vi "resonant.image queue to disk and to display queue_MD.vi"() -> ()   [LabVIEW 2012]
uses:
  <vilib>/Utility/VariantDataType/Type.ctl
  Custom Controls/file format type def.ctl
  GFG/GFGnumericGet.vi
  GFG/GFGbooleanGet.vi
  GFG/GFGstringGet.vi
  save images/save channels to raw bin files.vi
  save images/save channels to interleaved multi-tiff files.vi
  save images/save channels to separate multi-tiff files.vi
  save images/save channels to stacked multi-tiff files.vi
  save images/save channels to interleaved tiff series.vi
  save images/save channels to separate tiff series.vi
  save images/save channels to stacked tiff series.vi
  GFG/GFG library.lvlib
  <vilib>/Utility/VariantDataType/VariantType.lvlib
panel:
  out "element":i32
  out "error out 5":errorcluster
  out "size(s)":i32[](array[numeric])
  out "x/y":dbl
  out "error out 4":errorcluster
  out "error out 3":errorcluster
  out "error out 2":errorcluster
  out "# elements in image data queue":i32
  out "error out":errorcluster
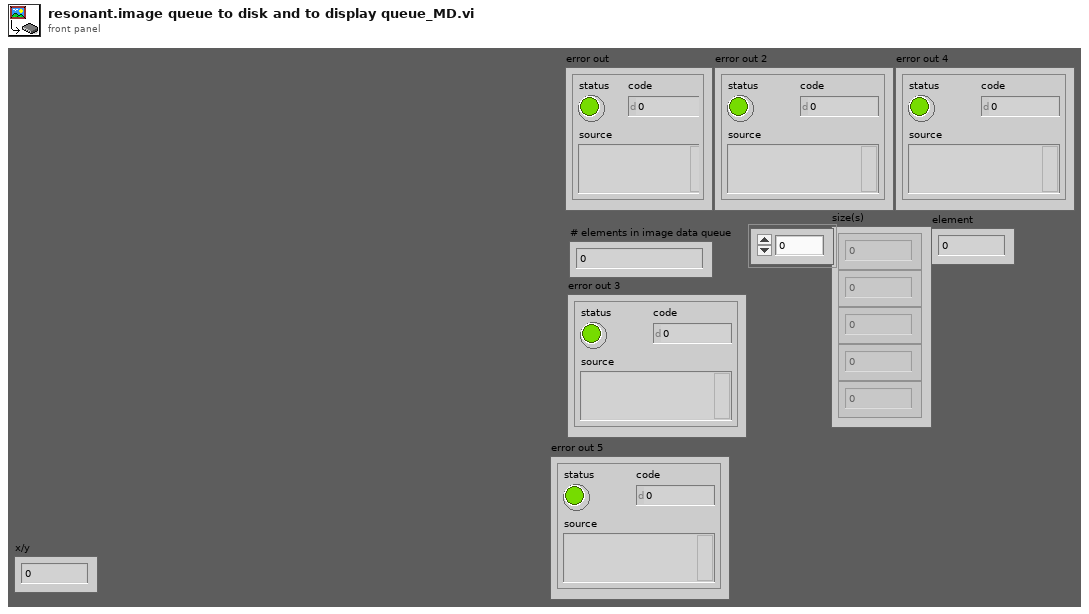
[diagram p1: front panel]
types:
  T1 = typedef "file format type def.ctl" = enum16{"16bit raw", "32bit raw", "16bit multi-tiff (interleave)", "16bit multi-tiff (separate)", "16bit multi-tiff (stacked)", "32bit multi-tiff (interleave)", "32bit multi-tiff (separate)", "32bit multi-tiff (stacked)", "16bit tiff series (interleave)", "16bit tiff series (separate)", "16bit tiff series (stacked)", "32bit tiff series (interleave)", "32bit tiff series (separate)", "32bit tiff series (stacked)"}
  T2 = cluster{"NewVal":bool, "Event Registration Refnum":refnum<event-registration>}
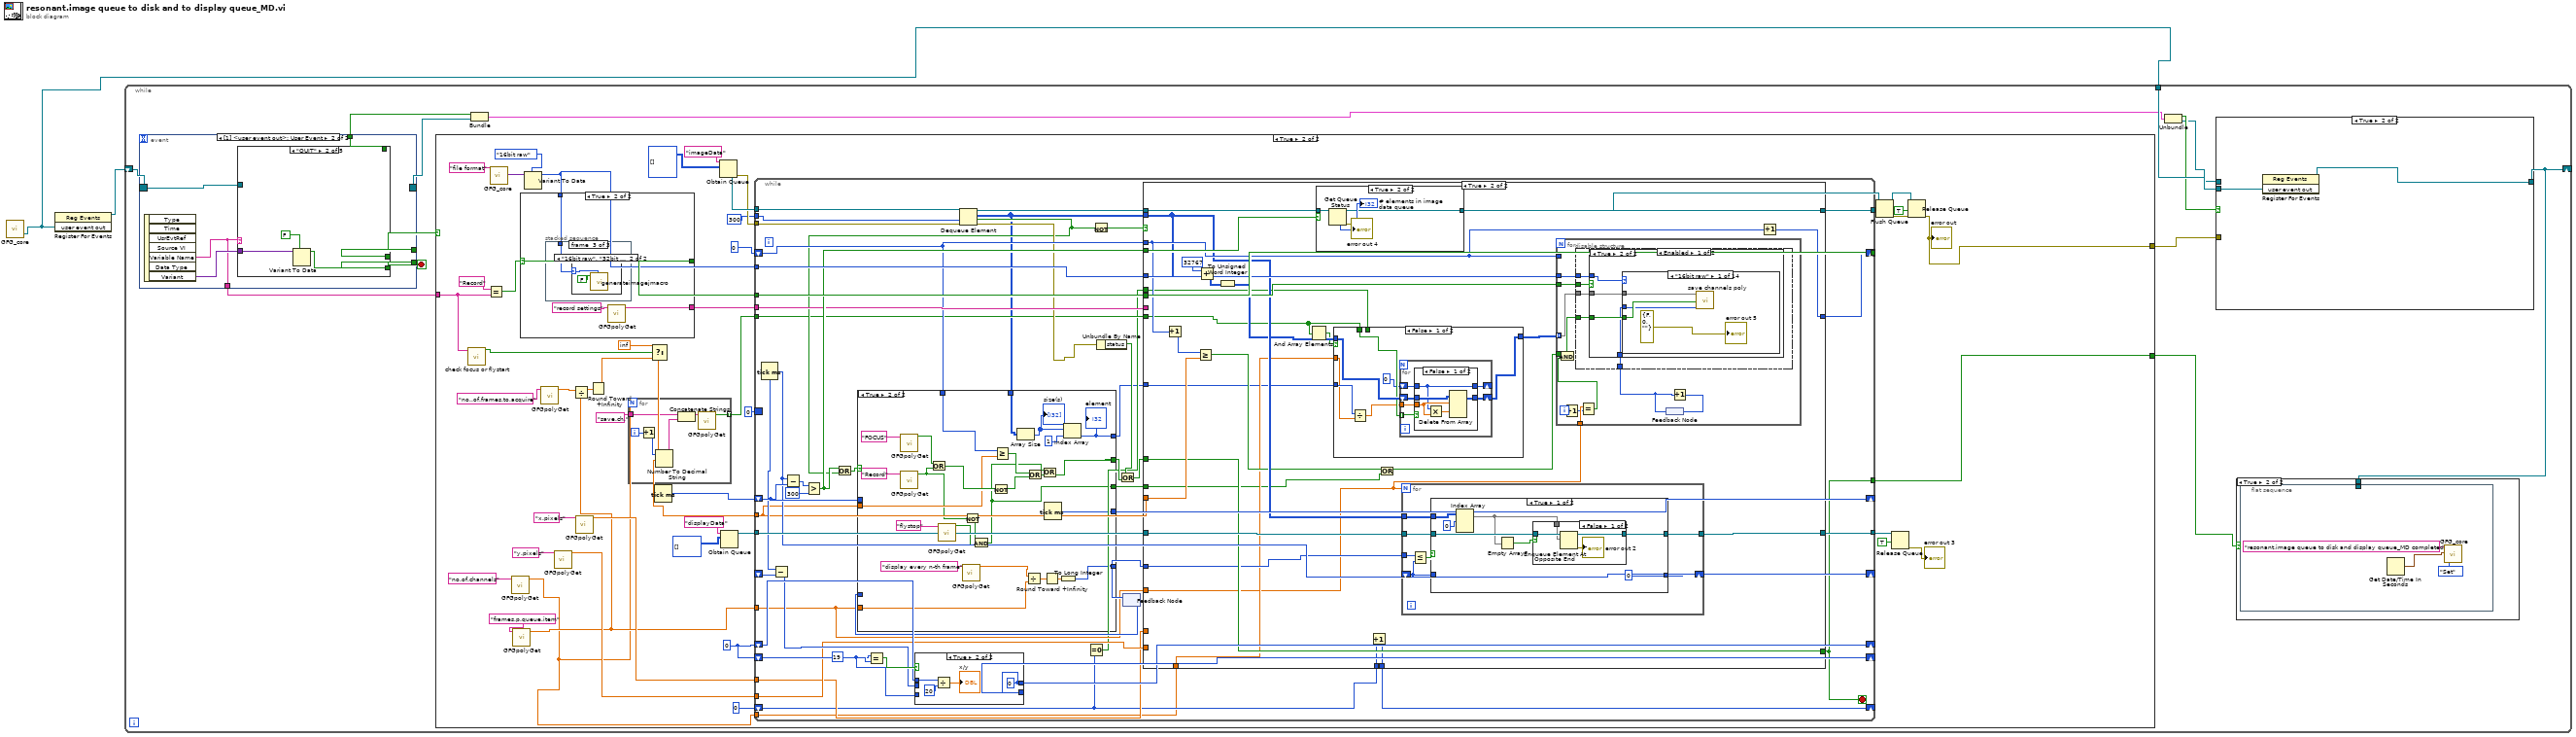
[diagram p0: block diagram]
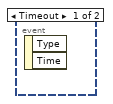
[diagram p4: hidden frame]
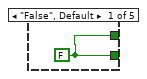
[diagram p5: hidden frame]
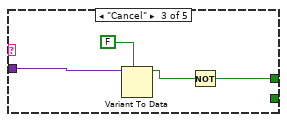
[diagram p6: hidden frame]
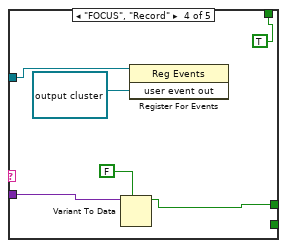
[diagram p7: hidden frame]
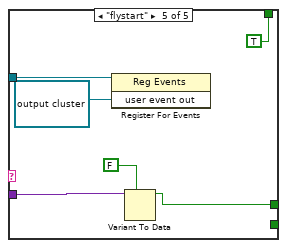
[diagram p8: hidden frame]
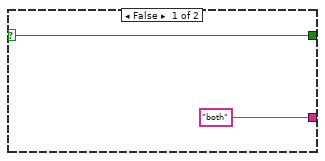
[diagram p10: hidden frame]
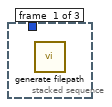
[diagram p11: hidden frame]
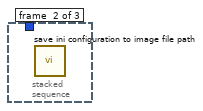
[diagram p12: hidden frame]
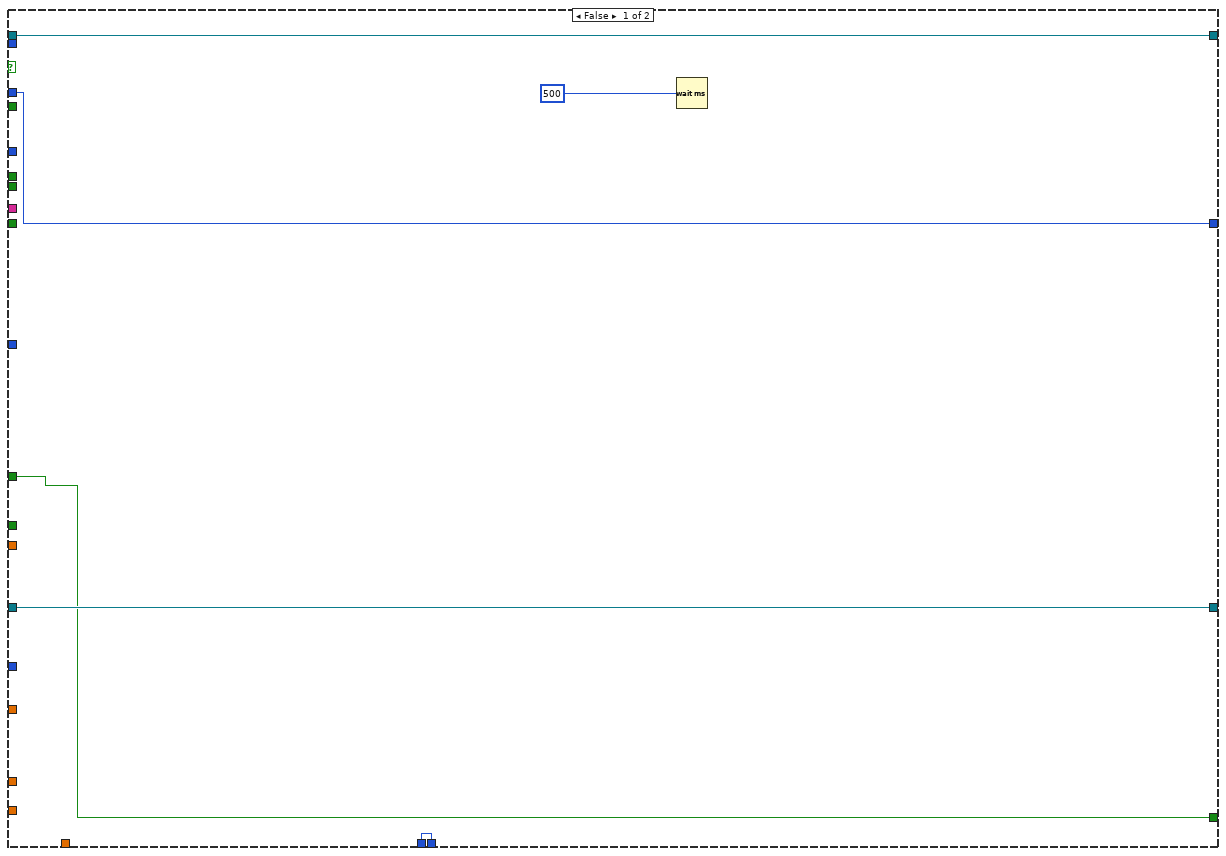
[diagram p14: hidden frame]
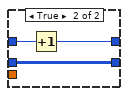
[diagram p15: hidden frame]
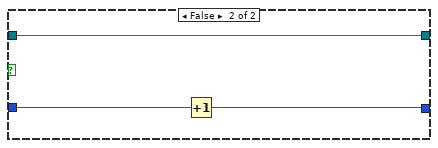
[diagram p18: hidden frame]
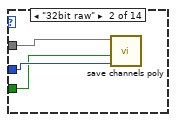
[diagram p20: hidden frame]
diagram:
  n1 = call "GFG_core.vi"() -> ("user event out"=w1:refnum<user-event>)  [unwired: 13 in, 6 out]
  n2 = register-events(w1) -> (reference out=w2:refnum<event-registration>)  [unwired: 2 in, 1 out]
  n3 = while {
    shift-right: [w4] -> _
    shift-left: w2 -> [w12]
    tunnel: w1 -> [w11]
    stop <- w14 stop-if-true
    n4 = event shown="[1] <user event out>: User Event" {
      selector: w12 -> [_ w24]
      dyn-events: [_ _] -> w8
      timeout: _ -> [_ _]
      tunnel: [_ w28] -> w15
      tunnel: [_ w27] -> w14
      tunnel: [_ w25] -> w13
      tunnel: [_ w23] -> w9
      event Timeout {
        n5 = event-data() -> ()  [unwired: 1 in, 2 out]
      }
      event User Event {
        n6 = event-data() -> ("Variable Name"=w25:string, "Variant"=w26:variant)  [unwired: 1 in, 5 out]
        n7 = case shown="\"QUIT\"" w25 {
          tunnel: [w29 _ w33 w40 w46] -> w28
          tunnel: [w29 w30 _ _ _] -> w27
          tunnel: w26 -> [_ w32 w35 w41 w47]
          tunnel: w24 -> [_ _ _ w38 w44]
          tunnel: [_ _ _ TRUE ("NewVal") TRUE ("NewVal")] -> w23
          frame "False", Default {
            w29 = FALSE ("NewVal")
          }
          frame "QUIT" {
            n8 = Variant To Data(type=FALSE ("NewVal"), Variant=w32) -> (data=w30:bool)  [unwired: 1 in, 1 out]
          }
          frame "Cancel" {
            n9 = Variant To Data(type=FALSE ("NewVal"), Variant=w35) -> (data=w34:bool)  [unwired: 1 in, 1 out]
            n10 = Not(x=w34) -> (.not. x?=w33:bool)
          }
          frame "FOCUS", "Record" {
            n11 = Variant To Data(type=FALSE ("NewVal"), Variant=w41) -> (data=w40:bool)  [unwired: 1 in, 1 out]
            n12 = register-events(reference=w38, refnum<user-event> refnum ("user event out")) -> ()  [unwired: 1 in, 2 out]
          }
          frame "flystart" {
            n13 = register-events(reference=w44, refnum<user-event> refnum ("user event out")) -> ()  [unwired: 1 in, 2 out]
            n14 = Variant To Data(type=FALSE ("NewVal"), Variant=w47) -> (data=w46:bool)  [unwired: 1 in, 1 out]
          }
        }
      }
    }
    n15 = case shown="True" w15 {
      tunnel: w13 -> [_ w66]
      tunnel: [_ w77] -> w10
      tunnel: [_ w61] -> w3
      frame False {
      }
      frame True {
        w79 = u32 0 ("millisecond timer value")
        n16 = call "check focus or flystart.vi"("x"=w66) -> ("x .or. y?"=w65:bool)  [unwired: 10 in]
        n17 = Equal?(x="Record", y=w66) -> (x = y?=w84:bool)
        n18 = call "GFG_core.vi"("Variable Name in"="file format") -> ("Variant Out"=w86:variant)  [unwired: 12 in, 6 out]
        n19 = call-poly "GFGpolyGet.vi"("Variable Name in"="no.of.channels" ("Tag in")) -> ("Numeric"=w49:dbl)  [unwired: 9 in, 1 out]
        n20 = call-poly "GFGpolyGet.vi"("Variable Name in"="frames.p.queue.item" ("Tag in")) -> ("Numeric"=w54:dbl)  [unwired: 9 in, 1 out]
        n21 = Variant To Data(type=file_format_type_def."16bit raw" ("file format"), Variant=w86) -> (data=w82:T1)  [unwired: 1 in, 1 out]
        n22 = case shown="True" w84 {
          selector: w84 -> [w104 w108]
          tunnel: [w104 w108] -> w83
          tunnel: w82 -> [_ w107]
          tunnel: ["both" ("String") w105] -> w72
          frame False {
          }
          frame True {
            n23 = stacked-sequence {
              tunnel: w107 -> [_ _ w109]
              frame #0 {
                n24 = call "generate filepath.vi"() -> ()  [unwired: 12 in]
              }
              frame #1 {
                n25 = call "save ini configuration to image file path.vi"() -> ()  [unwired: 12 in]
              }
              frame #2 {
                n26 = case shown="\"16bit raw\", \"32bit raw\"" w109 {
                  selector: w109 -> [_ w111]
                  frame Default {
                  }
                  frame "16bit raw", "32bit raw" {
                    n27 = call "generateimagejmacro.vi"("file format"=w111, "T:galvo F:resonant default:T"=FALSE) -> ()  [unwired: 10 in]
                  }
                }
              }
            }
            n28 = call-poly "GFGpolyGet.vi"("Variable Name in"="record settings" ("Tag in")) -> ("String"=w105:string)  [unwired: 10 in]
          }
        }
        n29 = call-poly "GFGpolyGet.vi"("Variable Name in"="no..of.frames.to.acquire" ("Tag in")) -> ("Numeric"=w74:dbl)  [unwired: 9 in, 1 out]
        n30 = call-poly "GFGpolyGet.vi"("Variable Name in"="y.pixels" ("Tag in")) -> ("Numeric"=w69:dbl)  [unwired: 9 in, 1 out]
        n31 = Divide(x=w74, y=w54) -> (x/y=w55:dbl)
        n32 = call-poly "GFGpolyGet.vi"("Variable Name in"="x.pixels" ("Tag in")) -> ("Numeric"=w68:dbl)  [unwired: 9 in, 1 out]
        n33 = Round Toward +Infinity(x=w55) -> (ceil(x): smallest int >= x=w53:dbl)
        n34 = for {
          N: w49 -> [_]
          tunnel: "save.ch." ("Variable Name in") -> [w102]
          tunnel: [w101] -> w50 mode=indexing
          i -> [w100]
          n35 = Increment(x=w100) -> (x+1=w99:i32)
          n36 = Number To Decimal String(number=w99) -> (decimal integer string=w97:string)  [unwired: 1 in]
          n37 = Concatenate Strings(w102, w97) -> (w98:string)
          n38 = call-poly "GFGpolyGet.vi"("Variable Name in"=w98) -> ("Boolean"=w101:bool)  [unwired: 10 in]
        }
        n39 = Select(t=inf, s=w65, f=w53) -> (s? t:f=w73:dbl)
        n40 = Tick Count (ms)() -> (millisecond timer value=w81:u32)
        n41 = Obtain Queue(name (unnamed)="imageData", element data type=i16[][][] [] ("initialized array")) -> (queue out=w89:refnum<queue>, error out=w67:errorcluster)  [unwired: 3 in, 1 out]
        n42 = Obtain Queue(name (unnamed)="displayData", element data type=i16[][] [] ("initialized array")) -> (queue out=w95:refnum<queue>)  [unwired: 3 in, 2 out]
        n43 = while {
          tunnel: [w155] -> w93
          tunnel: w95 -> [w158]
          tunnel: [w159] -> w94
          tunnel: w73 -> [w123]
          tunnel: w89 -> [w157]
          tunnel: w83 -> [w153]
          tunnel: w82 -> [w154]
          tunnel: [w153] -> _
          shift-right: [w150] -> _
          shift-left: w81 -> [w149]
          shift-right: [w142] -> _
          shift-left: w79 -> [w143]
          shift-right: [w144] -> _
          shift-left: w79 -> [w145]
          shift-right: [w141] -> _
          shift-left: _ -> [w139]
          tunnel: [w134] -> w61
          tunnel: w72 -> [w138]
          tunnel: w69 -> [w137]
          tunnel: w68 -> [w136]
          tunnel: w67 -> [w135]
          shift-right: [w131] -> _
          shift-left: u32 0 ("millisecond timer value") -> [w132]
          tunnel: 300 ("timeout in ms (-1)") -> [w124]
          tunnel: w54 -> [w120]
          tunnel: w50 -> [w119]
          shift-right: [w118] -> _
          shift-left: u32 0 ("millisecond timer value") -> [w117]
          tunnel: w49 -> [w115]
          border: 0 -> [_]
          stop <- w134 stop-if-true
          n44 = Tick Count (ms)() -> (millisecond timer value=w141:u32)
          n45 = Subtract(x=w141, y=w139) -> (x-y=w140:u32)
          n46 = Subtract(x=w141, y=w149) -> (x-y=w152:u32)
          n47 = Greater?(x=w152, y=u32 300) -> (0:w148:bool)
          n48 = Equal?(x=w145, y=u32 19) -> (x = y?=w146:bool)
          n49 = case shown="True" w146 {
            tunnel: w140 -> [w311 _]
            tunnel: [w310 w313] -> w142
            tunnel: w143 -> [w309 w312]
            tunnel: w145 -> [w308 _]
            tunnel: [w307 w313] -> w144
            frame False {
              n50 = Increment(x=w308) -> (x+1=w307:u32)
              n51 = Add(x=w309, y=w311) -> (x+y=w310:u32)
            }
            frame True {
              w313 = u32 0
              n52 = Divide(x=w312, y=u32 20) -> (x/y=→"x/y":dbl)
            }
          }
          n53 = Dequeue Element(queue=w157, timeout in ms (-1)=w124, error in (no error)=w135) -> (queue out=w156:refnum<queue>, element=w114:i16[][][], timed out?=w125:bool, error out=w130:errorcluster)
          n54 = Or(x=w148, y=w125) -> (x .or. y?=w126:bool)
          n55 = Equal To 0?(x=w117) -> (x = 0?=w116:bool)
          n56 = Not(x=w125) -> (.not. x?=w133:bool)
          n57 = Unbundle By Name(w130) -> ("status"=w128:bool)
          n58 = feedback #1() -> (w122:i32)  [unwired: 1 in]
          n59 = case shown="True" w126 {
            tunnel: [_ w331] -> w129
            tunnel: w132 -> [_ w320]
            tunnel: [w318 w341] -> w150
            tunnel: w149 -> [w318 _]
            tunnel: w123 -> [_ w337]
            tunnel: [w317 w327] -> w121
            tunnel: w120 -> [_ w325]
            tunnel: w122 -> [w317 _]
            tunnel: w114 -> [_ w323]
            tunnel: [w316 w321] -> w113
            tunnel: [_ w319] -> w112
            frame False {
              n60 = local read "element"() -> (w316:i32)
            }
            frame True {
              n61 = call-poly "GFGpolyGet.vi"("Variable Name in"="FOCUS") -> ("Boolean"=w342:bool)  [unwired: 10 in]
              n62 = call-poly "GFGpolyGet.vi"("Variable Name in"="Record") -> ("Boolean"=w332:bool)  [unwired: 10 in]
              n63 = Or(x=w342, y=w332) -> (x .or. y?=w340:bool)
              n64 = call-poly "GFGpolyGet.vi"("Variable Name in"="flystop") -> ("Boolean"=w333:bool)  [unwired: 10 in]
              n65 = call-poly "GFGpolyGet.vi"("Variable Name in"="display every n-th frame" ("Tag in")) -> ("Numeric"=w329:dbl)  [unwired: 9 in, 1 out]
              n66 = Not(x=w332) -> (.not. x?=w334:bool)
              n67 = And(x=w334, y=w333) -> (x .and. y?=w319:bool)
              n68 = Not(x=w340) -> (.not. x?=w338:bool)
              n69 = Greater Or Equal?(x=w320, y=w337) -> (x >= y?=w339:bool)
              n70 = Array Size(array=w323) -> (size(s)=w322:i32[])
              "size(s)" <- w322
              n71 = Divide(x=w329, y=w325) -> (x/y=w328:dbl)
              n72 = Or(x=w339, y=w338) -> (x .or. y?=w336:bool)
              n73 = Or(x=w319, y=w336) -> (x .or. y?=w331:bool)
              n74 = Round Toward +Infinity(x=w328) -> (ceil(x): smallest int >= x=w326:dbl)
              n75 = Tick Count (ms)() -> (millisecond timer value=w341:u32)
              n76 = To Long Integer(number=w326) -> (32bit integer=w327:i32)
              n77 = Index Array(array=w322, index=1) -> (element=w321:i32)
              "element" <- w321
            }
          }
          n78 = Or(x=w128, y=w129) -> (x .or. y?=w127:bool)
          n79 = feedback-in #1(w121) -> ()
          n80 = case shown="True" w133 {
            tunnel: [w164 w194] -> w159
            tunnel: w158 -> [w164 w193]
            tunnel: w156 -> [w165 w192]
            tunnel: [w165 w191] -> w155
            tunnel: w154 -> [_ w190]
            tunnel: w153 -> [_ w189]
            tunnel: w148 -> [_ w188]
            tunnel: w132 -> [w163 w184]
            tunnel: w114 -> [_ w179]
            tunnel: w138 -> [_ _]
            tunnel: w137 -> [_ _]
            tunnel: w136 -> [_ _]
            tunnel: w127 -> [w161 w182]
            tunnel: [w161 w182] -> w134
            tunnel: [w163 w186] -> w131
            tunnel: w123 -> [_ w185]
            tunnel: w121 -> [_ w181]
            tunnel: w120 -> [_ w169]
            tunnel: w119 -> [_ w176]
            tunnel: w116 -> [_ w174]
            tunnel: w117 -> [w160 w173]
            tunnel: [w160 w172] -> w118
            tunnel: w115 -> [_ w171]
            tunnel: w113 -> [_ w170]
            tunnel: w112 -> [_ w167]
            frame False {
              n81 = Wait (ms)(milliseconds to wait=u32 500) -> ()  [unwired: 1 out]
            }
            frame True {
              n82 = Increment(x=w184) -> (x+1=w183:u32)
              n83 = Greater Or Equal?(x=w183, y=w185) -> (x >= y?=w175:bool)
              n84 = Add(x=i16 32767, y=w179) -> (x+y=w180:i16[][][])
              n85 = To Unsigned Word Integer(number=w180) -> (unsigned 16bit integer=w178:u16[][][])
              n86 = And Array Elements(Boolean array=w176) -> (logical AND=w166:bool)
              n87 = case shown="True" w188 {
                tunnel: w192 -> [w302 w305]
                tunnel: [w302 w304] -> w191
                frame False {
                }
                frame True {
                  n88 = Get Queue Status(queue=w305) -> (queue out=w304:refnum<queue>, error out=→"error out 4":errorcluster, # elements in queue=→"# elements in image data queue":i32)  [unwired: 2 in, 5 out]
                }
              }
              n89 = case shown="False" w166 {
                tunnel: w174 -> [_ _]
                tunnel: w178 -> [w201 w216]
                tunnel: [w200 w216] -> w187
                tunnel: w171 -> [w197 _]
                tunnel: w176 -> [w199 _]
                tunnel: w170 -> [w198 _]
                frame False {
                  n90 = Divide(x=w198, y=w197) -> (x/y=w196:dbl)
                  n91 = for {
                    tunnel: w199 -> [w203] mode=indexing
                    shift-right: [w204] -> w200
                    shift-left: w201 -> [w207]
                    tunnel: w196 -> [w205]
                    shift-right: [w202] -> _
                    shift-left: 0 ("index") -> [w206]
                    n92 = case shown="False" w203 {
                      tunnel: w207 -> [w212 w215]
                      tunnel: w206 -> [w208 w214]
                      tunnel: w205 -> [w210 _]
                      tunnel: [w209 w215] -> w204
                      tunnel: [w208 w213] -> w202
                      frame False {
                        n93 = Multiply(x=w208, y=w210) -> (x*y=w211:dbl)
                        n94 = Delete From Array(array=w212, length=w210, index (dim 1)=w211) -> (array with subset deleted=w209:u16[][][])  [unwired: 2 in, 1 out]
                      }
                      frame True {
                        n95 = Increment(x=w214) -> (x+1=w213:i32)
                      }
                    }
                  }
                }
                frame True {
                }
              }
              n96 = Increment(x=w173) -> (x+1=w172:u32)
              n97 = Or(x=w175, y=w167) -> (x .or. y?=w168:bool)
              n98 = for {
                N: w169 -> [_]
                tunnel: [w223] -> w194
                tunnel: w193 -> [w222]
                tunnel: w179 -> [w221]
                shift-right: [w220] -> _
                shift-left: _ -> [w217]
                tunnel: w181 -> [w219]
                n99 = Less Or Equal?(x=w219, y=w217) -> (x <= y?=w218:bool)
                n100 = case shown="True" w218 {
                  tunnel: [w230 w238] -> w223
                  tunnel: w222 -> [w229 w238]
                  tunnel: w221 -> [w227 _]
                  tunnel: [0 w236] -> w220
                  tunnel: w217 -> [_ w237]
                  frame True {
                    n101 = Index Array(array=w227, index (dim 0)=0 ("index (page)")) -> (element=w224:i16[][])  [unwired: 2 in]
                    n102 = Empty Array?(array=w224) -> (empty?=w228:bool)
                    n103 = case shown="False" w228 {
                      tunnel: [w234 w235] -> w230
                      tunnel: w229 -> [w233 w235]
                      tunnel: w224 -> [w231 _]
                      frame False {
                        n104 = Enqueue Element At Opposite End(queue=w233, element=w231) -> (queue out=w234:refnum<queue>, error out=→"error out 2":errorcluster)  [unwired: 2 in, 1 out]
                      }
                      frame True {
                      }
                    }
                  }
                  frame False {
                    n105 = Increment(x=w237) -> (x+1=w236:i32)
                  }
                }
              }
              n106 = for {
                tunnel: w190 -> [w249]
                tunnel: w189 -> [w248]
                tunnel: w187 -> [w247] mode=indexing
                tunnel: w184 -> [_]
                tunnel: w168 -> [w246]
                tunnel: w169 -> [w244]
                i -> [w245]
                n107 = Increment(x=w245) -> (x+1=w241:i32)
                n108 = Equal?(x=w244, y=w241) -> (x = y?=w242:bool)
                n109 = And(x=w246, y=w242) -> (x .and. y?=w243:bool)
                n110 = feedback #2() -> (w239:i32)
                n111 = disable-structure shown="Enabled" {
                  disable-tunnel: w249 -> [w254 _]
                  disable-tunnel: w248 -> [w253 _]
                  disable-tunnel: w247 -> [w252 _]
                  disable-tunnel: w243 -> [w251 _]
                  disable-tunnel: w239 -> [w250 _]
                  frame Enabled {
                    n112 = case shown="True" w253 {
                      tunnel: w251 -> [_ w257]
                      tunnel: w254 -> [_ w256]
                      tunnel: w252 -> [_ w258]
                      tunnel: w250 -> [_ w255]
                      frame False {
                      }
                      frame True {
                        n113 = case shown="\"16bit raw\"" w256 {
                          tunnel: w258 -> [w262 w265 w268 w271 w274 w277 w280 w283 w286 w289 w292 w295 w298 w301]
                          tunnel: w255 -> [w259 w264 w267 w270 w273 w276 w279 w282 w285 w288 w291 w294 w297 w300]
                          tunnel: w257 -> [w261 w263 w266 w269 w272 w275 w278 w281 w284 w287 w290 w293 w296 w299]
                          frame "16bit raw" {
                            n114 = call-poly "save channels poly.vi"("frame number in"=w259, "last frame"=w261, "image data in (U16)"=w262) -> ()  [unwired: 9 in]
                            "error out 5" <- errorcluster {"status"=FALSE, "code"=0, "source"=""} ("error out 4")
                          }
                          frame "32bit raw" {
                            n115 = call-poly "save channels poly.vi"("frame number in"=w264, "last frame"=w263, "image data in (U16)"=w265) -> ()  [unwired: 9 in]
                          }
                          frame "16bit multi-tiff (interleave)" {
                            n116 = call-poly "save channels poly.vi"("frame number in"=w267, "last frame"=w266, "image data in"=w268) -> ()  [unwired: 9 in]
                          }
                          frame "16bit multi-tiff (separate)" {
                            n117 = call-poly "save channels poly.vi"("frame number in"=w270, "last frame"=w269, "image data in"=w271) -> ()  [unwired: 9 in]
                          }
                          frame "16bit multi-tiff (stacked)" {
                            n118 = call-poly "save channels poly.vi"("frame number in"=w273, "last frame"=w272, "image data in"=w274) -> ()  [unwired: 9 in]
                          }
                          frame "32bit multi-tiff (interleave)" {
                            n119 = call-poly "save channels poly.vi"("frame number in"=w276, "last frame"=w275, "image data in"=w277) -> ()  [unwired: 9 in]
                          }
                          frame "32bit multi-tiff (separate)" {
                            n120 = call-poly "save channels poly.vi"("frame number in"=w279, "last frame"=w278, "image data in"=w280) -> ()  [unwired: 9 in]
                          }
                          frame "32bit multi-tiff (stacked)" {
                            n121 = call-poly "save channels poly.vi"("frame number in"=w282, "last frame"=w281, "image data in"=w283) -> ()  [unwired: 9 in]
                          }
                          frame "16bit tiff series (interleave)" {
                            n122 = call-poly "save channels poly.vi"("frame number in"=w285, "last frame"=w284, "image data in"=w286) -> ()  [unwired: 9 in]
                          }
                          frame "16bit tiff series (separate)" {
                            n123 = call-poly "save channels poly.vi"("frame number in"=w288, "last frame"=w287, "image data in"=w289) -> ()  [unwired: 9 in]
                          }
                          frame "16bit tiff series (stacked)" {
                            n124 = call-poly "save channels poly.vi"("frame number in"=w291, "last frame"=w290, "image data in"=w292) -> ()  [unwired: 9 in]
                          }
                          frame "32bit tiff series (interleave)" {
                            n125 = call-poly "save channels poly.vi"("frame number in"=w294, "last frame"=w293, "image data in"=w295) -> ()  [unwired: 9 in]
                          }
                          frame "32bit tiff series (separate)" {
                            n126 = call-poly "save channels poly.vi"("frame number in"=w297, "last frame"=w296, "image data in"=w298) -> ()  [unwired: 9 in]
                          }
                          frame "32bit tiff series (stacked)" {
                            n127 = call-poly "save channels poly.vi"("frame number in"=w300, "last frame"=w299, "image data in"=w301) -> ()  [unwired: 9 in]
                          }
                        }
                      }
                    }
                  }
                  frame Disabled {
                  }
                }
                n128 = Increment(x=w239) -> (x+1=w240:i32)
                n129 = feedback-in #2(w240) -> ()
              }
              n130 = Increment(x=w184) -> (x+1=w186:u32)
            }
          }
        }
        n131 = Flush Queue(queue=w93) -> (queue out=w92:refnum<queue>, error out=w91:errorcluster)  [unwired: 1 in, 1 out]
        n132 = Release Queue(queue=w94, force destroy? (F)=TRUE) -> (error out=→"error out 3":errorcluster)  [unwired: 1 in, 2 out]
        n133 = Release Queue(queue=w92, force destroy? (F)=TRUE, error in (no error)=w91) -> (error out=w77:errorcluster)  [unwired: 2 out]
        "error out" <- w77
      }
    }
    n134 = Bundle("NewVal"=w9, "Event Registration Refnum"=w8) -> (w7:T2)  [unwired: 1 in]
    n135 = Unbundle(w7) -> ("NewVal"=w6:bool, "Event Registration Refnum"=w5:refnum<event-registration>)
    n136 = case shown="True" w6 {
      tunnel: [w20 w22] -> w4
      tunnel: w11 -> [_ w21]
      tunnel: w10 -> [_ _]
      tunnel: w5 -> [w20 _]
      frame False {
      }
      frame True {
        n137 = register-events(w21) -> (reference out=w22:refnum<event-registration>)  [unwired: 2 in, 1 out]
      }
    }
    n138 = case shown="True" w3 {
      tunnel: w4 -> [_ w16]
      frame False {
      }
      frame True {
        n139 = flat-sequence {
          tunnel: w16 -> [_]
          frame #0 {
            n140 = Get Date/Time In Seconds() -> (seconds since 1Jan1904=w17:timestamp)
            n141 = call "GFG_core.vi"("Variable Name in"="resonant.image queue to disk and display queue_MD completed", "Variant in"=w17, "Action"=enum16{"Init", "Set", "Get"}."Set") -> ()  [unwired: 10 in, 7 out]
          }
        }
      }
    }
  }
